vi "One_point_Auto-corr.vi"(5 "Delta T":dbl format="%.2f", 7 "No of products in":i32[](array[numeric]), 8 "Auto-corr in":dbl[](array[numeric]) format="%.2f", 9 "Total Arr times":dbl[](array[numeric]) format="%.2f", 10 "U":dbl[](array[numeric]) format="%.2f") -> (0 "No of products out":i32[](array[numeric]), 1 "Auto-corr out":dbl[](array[numeric]) format="%.2f")   [LabVIEW 2010]
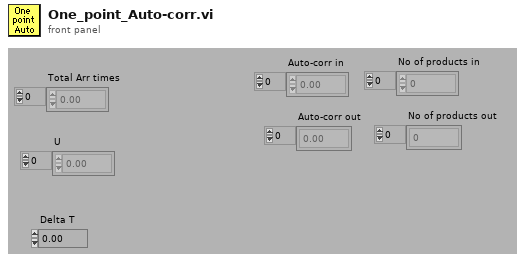
[diagram p1: front panel]
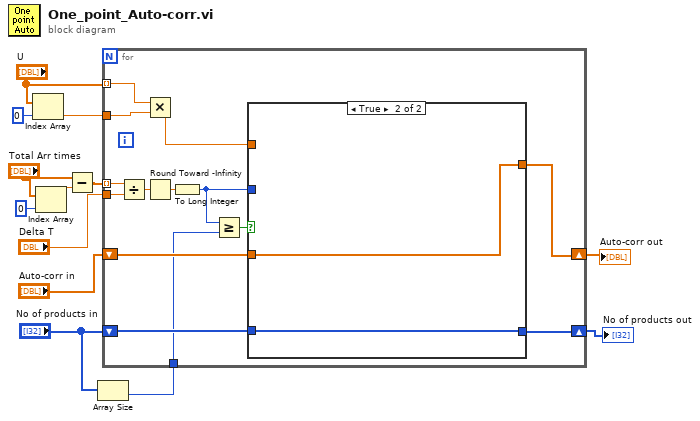
[diagram p0: block diagram]
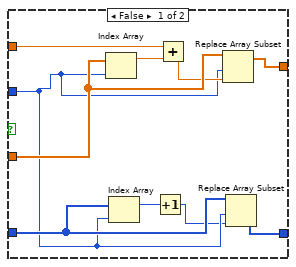
[diagram p2: hidden frame]
diagram:
  n1 = Index Array(array="U", index=0) -> (element=w12:dbl)
  n2 = Index Array(array="Total Arr times", index=0) -> (element=w9:dbl)
  n3 = Subtract(x="Total Arr times", y=w9) -> (x-y=w7:dbl[])
  n4 = Array Size(array="No of products in") -> (size(s)=w1:i32)
  n5 = for {
    shift-right: [w19] -> w3
    shift-left: "Auto-corr in" -> [w20]
    tunnel: w12 -> [w27]
    tunnel: "U" -> [w26] mode=indexing
    tunnel: w7 -> [w25] mode=indexing
    tunnel: "Delta T" -> [w24]
    shift-right: [w17] -> w4
    shift-left: "No of products in" -> [w18]
    tunnel: w1 -> [w15]
    n6 = Divide(x=w25, y=w24) -> (x/y=w23:dbl)
    n7 = Multiply(x=w26, y=w27) -> (x*y=w21:dbl)
    n8 = Round Toward -Infinity(1:w23) -> (0:w22:dbl)
    n9 = To Long Integer(number=w22) -> (32bit integer=w14:i32)
    n10 = Greater Or Equal?(x=w14, y=w15) -> (x >= y?=w16:bool)
    n11 = case shown="True" w16 {
      tunnel: w21 -> [w36 _]
      tunnel: w20 -> [w35 w39]
      tunnel: [w33 w39] -> w19
      tunnel: w18 -> [w32 w38]
      tunnel: [w31 w38] -> w17
      tunnel: w14 -> [w30 _]
      frame False {
        n12 = Index Array(array=w35, index=w30) -> (element=w37:dbl)
        n13 = Index Array(array=w32, index=w30) -> (element=w29:i32)
        n14 = Increment(x=w29) -> (x+1=w28:i32)
        n15 = Add(x=w36, y=w37) -> (x+y=w34:dbl)
        n16 = Replace Array Subset(array=w35, new element=w34, index=w30) -> (w33:dbl[])
        n17 = Replace Array Subset(array=w32, new element=w28, index=w30) -> (w31:i32[])
      }
      frame True {
      }
    }
  }
  "Auto-corr out" <- w3
  "No of products out" <- w4
